vi "Query (Dynamic) 2.vi"(5 "Use VISA? (not visa GPIB only)":bool, 6 "Path Only":bool, 7 "Comms Layer":T1, 8 "error in":errorcluster, 9 "byte count":u32=4096 caption="byte count (4096)", 10 "Command":string, 11 "Comms":refnum<visa-resource-name>) -> (0 "error out":errorcluster, 2 "Response":string, 3 "Comms out":refnum<visa-resource-name>, 4 "path":path)   [LabVIEW 2013]
uses:
  <instrlib>/Mercury iXX/Public/Controls/Comms Transport Layer.ctl
  <vilib>/Instr/_visa.llb/VISA Flush IO Buffer Mask.ctl
  <instrlib>/Mercury iXX/Mercury iXX.lvlib
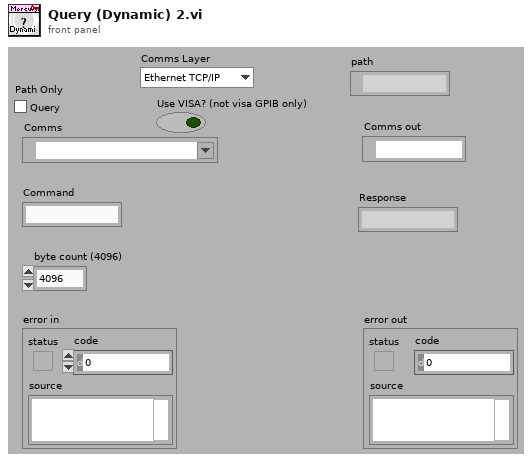
[diagram p1: front panel]
types:
  T1 = typedef "Mercury iXX.lvlib/Comms Transport Layer.ctl" = enum16{"Ethernet TCP/IP", "USB", "ISOBus - RS-232", "GPIB"}
  T2 = typedef "VISA Flush IO Buffer Mask.ctl" = u16
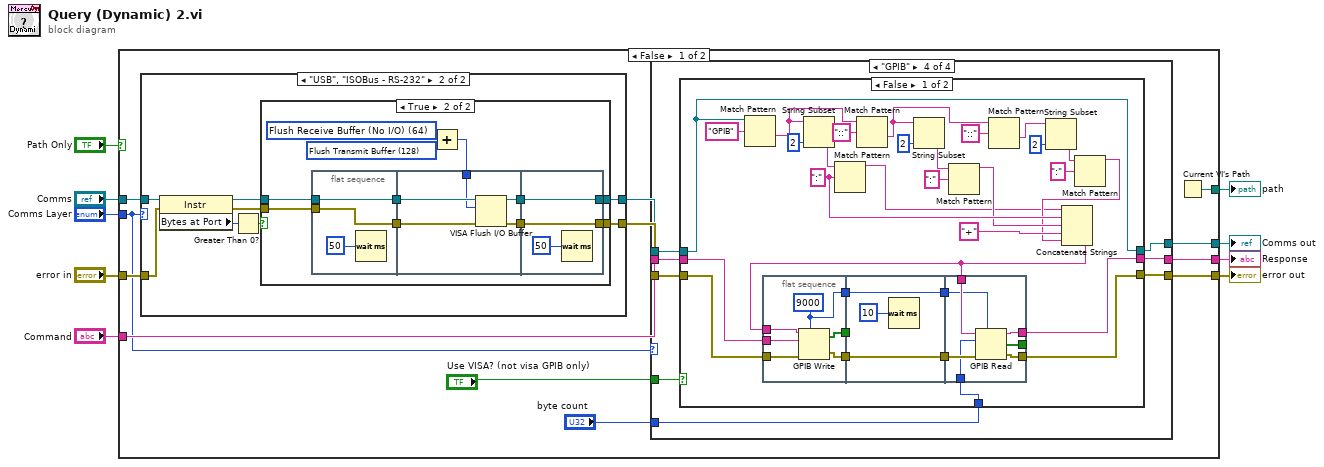
[diagram p0: block diagram]
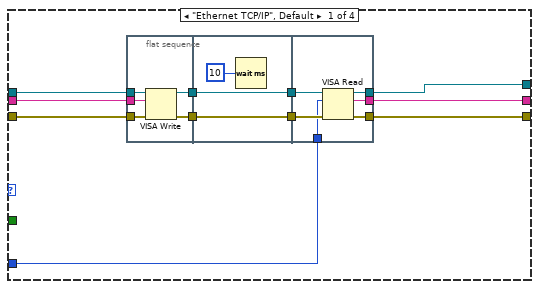
[diagram p2: hidden frame]
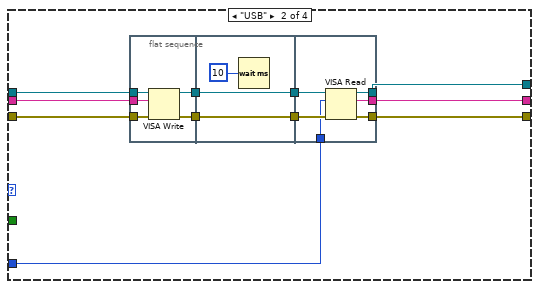
[diagram p3: hidden frame]
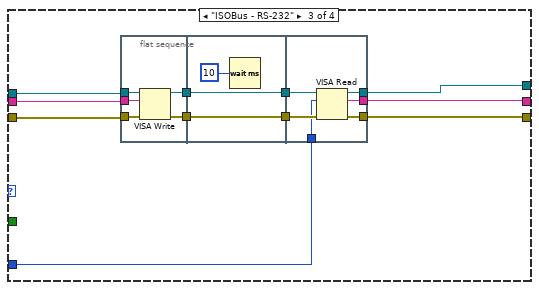
[diagram p4: hidden frame]
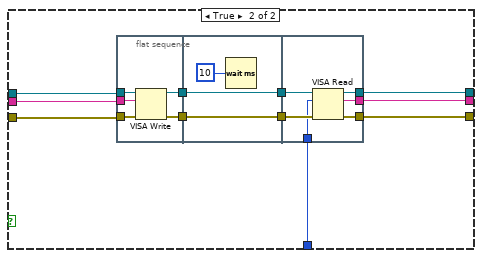
[diagram p5: hidden frame]
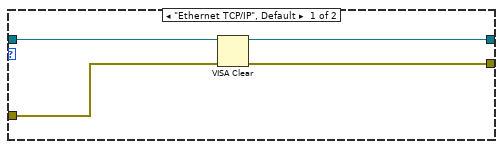
[diagram p6: hidden frame]
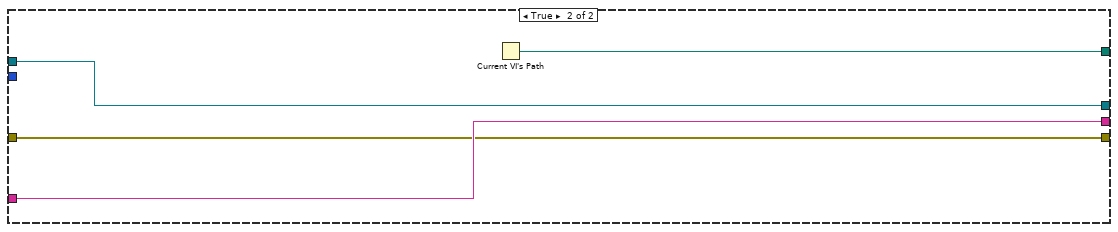
[diagram p8: hidden frame]
diagram:
  n1 = case shown="False" "Path Only" {
    tunnel: [w12 w215] -> w9
    tunnel: "Command" -> [w20 w215]
    tunnel: [w19 w216] -> w7
    tunnel: "error in" -> [w18 w214]
    tunnel: [w16 w214] -> w5
    tunnel: "Comms Layer" -> [w11 _]
    tunnel: "Comms" -> [w15 w216]
    tunnel: [w13 w213] -> w1
    frame False {
      n2 = case shown="\"USB\", \"ISOBus - RS-232\"" w11 {
        tunnel: w18 -> [w180 w187]
        tunnel: [w179 w181] -> w17
        tunnel: w15 -> [w178 w188]
        tunnel: [w177 w183] -> w14
        frame "Ethernet TCP/IP", Default {
          n3 = VISA Clear(VISA resource name=w178, error in (no error)=w180) -> (VISA resource name out=w177:refnum<visa-resource-name>, error out=w179:errorcluster)
        }
        frame "USB", "ISOBus - RS-232" {
          n4 = property class="Instr"(reference=w188, error in=w187) -> (reference out=w184:refnum<visa-resource-name>, error out=w182:errorcluster, "Bytes at Port"=w186:u32)
          n5 = Greater Than 0?(x=w186) -> (x > 0?=w185:bool)
          n6 = case shown="True" w185 {
            tunnel: w184 -> [w190 w199]
            tunnel: [w190 w201] -> w183
            tunnel: w182 -> [w189 w197]
            tunnel: [w189 w194] -> w181
            frame False {
            }
            frame True {
              w192 = T2 128 items=["Flush Receive Buffer"=16, "Write Transmit Buffer to Device"=32, "Flush Receive Buffer (No I/O)"=64, "Flush Transmit Buffer"=128] ("Mask")
              w193 = T2 64 items=["Flush Receive Buffer"=16, "Write Transmit Buffer to Device"=32, "Flush Receive Buffer (No I/O)"=64, "Flush Transmit Buffer"=128] ("Mask")
              n7 = flat-sequence {
                tunnel: w199 -> [w203]
                tunnel: [w203] -> w198
                tunnel: w197 -> [w202]
                tunnel: [w202] -> w196
                tunnel: [w209] -> w200
                tunnel: w198 -> [w208]
                tunnel: w196 -> [w207]
                tunnel: [w206] -> w195
                tunnel: w191 -> [w205]
                tunnel: [w211] -> w201
                tunnel: w200 -> [w211]
                tunnel: w195 -> [w210]
                tunnel: [w210] -> w194
                frame #0 {
                  n8 = Wait (ms)(milliseconds to wait=u32 50) -> ()  [unwired: 1 out]
                }
                frame #1 {
                  n9 = VISA Flush I/O Buffer(VISA resource name=w208, mask (16)=w205, error in (no error)=w207) -> (VISA resource name out=w209:refnum<visa-resource-name>, error out=w206:errorcluster)
                }
                frame #2 {
                  n10 = Wait (ms)(milliseconds to wait=u32 50) -> ()  [unwired: 1 out]
                }
              }
              n11 = Add(x=w193, y=w192) -> (x+y=w191:T2)
            }
          }
        }
      }
      n12 = case shown="\"GPIB\"" w11 {
        tunnel: "byte count" -> [w25 w53 w75 w101]
        tunnel: w20 -> [w27 w52 w77 w103]
        tunnel: [w22 w51 w72 w100] -> w19
        tunnel: w17 -> [w26 w50 w76 w102]
        tunnel: [w24 w49 w74 w98] -> w16
        tunnel: w14 -> [w28 w48 w78 w104]
        tunnel: [w23 w47 w73 w99] -> w12
        tunnel: "Use VISA? (not visa GPIB only)" -> [_ _ _ w97]
        frame "Ethernet TCP/IP", Default {
          n13 = flat-sequence {
            tunnel: w28 -> [w34]
            tunnel: w27 -> [w35]
            tunnel: [w37] -> w32
            tunnel: [w36] -> w31
            tunnel: w26 -> [w33]
            tunnel: w32 -> [w39]
            tunnel: w31 -> [w38]
            tunnel: [w39] -> w30
            tunnel: [w38] -> w29
            tunnel: w30 -> [w46]
            tunnel: w29 -> [w45]
            tunnel: [w44] -> w24
            tunnel: w25 -> [w43]
            tunnel: [w42] -> w22
            tunnel: [w41] -> w23
            frame #0 {
              n14 = VISA Write(VISA resource name=w34, write buffer=w35, error in (no error)=w33) -> (VISA resource name out=w37:refnum<visa-resource-name>, error out=w36:errorcluster)  [unwired: 1 out]
            }
            frame #1 {
              n15 = Wait (ms)(milliseconds to wait=u32 10) -> ()  [unwired: 1 out]
            }
            frame #2 {
              n16 = VISA Read(VISA resource name=w46, byte count=w43, error in (no error)=w45) -> (VISA resource name out=w42:refnum<visa-resource-name>, read buffer=w41:string, error out=w44:errorcluster)  [unwired: 1 out]
            }
          }
        }
        frame "USB" {
          n17 = flat-sequence {
            tunnel: w48 -> [w59]
            tunnel: w52 -> [w60]
            tunnel: [w62] -> w57
            tunnel: [w61] -> w56
            tunnel: w50 -> [w58]
            tunnel: w57 -> [w64]
            tunnel: w56 -> [w63]
            tunnel: [w64] -> w55
            tunnel: [w63] -> w54
            tunnel: w55 -> [w71]
            tunnel: w54 -> [w70]
            tunnel: [w69] -> w49
            tunnel: w53 -> [w68]
            tunnel: [w67] -> w51
            tunnel: [w66] -> w47
            frame #0 {
              n18 = VISA Write(VISA resource name=w59, write buffer=w60, error in (no error)=w58) -> (VISA resource name out=w62:refnum<visa-resource-name>, error out=w61:errorcluster)  [unwired: 1 out]
            }
            frame #1 {
              n19 = Wait (ms)(milliseconds to wait=u32 10) -> ()  [unwired: 1 out]
            }
            frame #2 {
              n20 = VISA Read(VISA resource name=w71, byte count=w68, error in (no error)=w70) -> (VISA resource name out=w67:refnum<visa-resource-name>, read buffer=w66:string, error out=w69:errorcluster)  [unwired: 1 out]
            }
          }
        }
        frame "ISOBus - RS-232" {
          n21 = flat-sequence {
            tunnel: w78 -> [w84]
            tunnel: w77 -> [w85]
            tunnel: [w87] -> w82
            tunnel: [w86] -> w81
            tunnel: w76 -> [w83]
            tunnel: w82 -> [w89]
            tunnel: w81 -> [w88]
            tunnel: [w89] -> w80
            tunnel: [w88] -> w79
            tunnel: w80 -> [w96]
            tunnel: w79 -> [w95]
            tunnel: [w94] -> w74
            tunnel: w75 -> [w93]
            tunnel: [w92] -> w72
            tunnel: [w91] -> w73
            frame #0 {
              n22 = VISA Write(VISA resource name=w84, write buffer=w85, error in (no error)=w83) -> (VISA resource name out=w87:refnum<visa-resource-name>, error out=w86:errorcluster)  [unwired: 1 out]
            }
            frame #1 {
              n23 = Wait (ms)(milliseconds to wait=u32 10) -> ()  [unwired: 1 out]
            }
            frame #2 {
              n24 = VISA Read(VISA resource name=w96, byte count=w93, error in (no error)=w95) -> (VISA resource name out=w92:refnum<visa-resource-name>, read buffer=w91:string, error out=w94:errorcluster)  [unwired: 1 out]
            }
          }
        }
        frame "GPIB" {
          n25 = case shown="False" w97 {
            tunnel: w104 -> [w123 w158]
            tunnel: w103 -> [w132 w157]
            tunnel: w102 -> [w131 w156]
            tunnel: [w123 w155] -> w100
            tunnel: [w130 w154] -> w99
            tunnel: [w118 w153] -> w98
            tunnel: w101 -> [w129 w152]
            frame False {
              w112 = ":" ("regular expression")
              n26 = Match Pattern(string=w123, regular expression="GPIB") -> (after substring=w125:string)  [unwired: 1 in, 3 out]
              n27 = flat-sequence {
                tunnel: [w141] -> w135
                tunnel: [w140] -> w134
                tunnel: w132 -> [w139]
                tunnel: w131 -> [w138]
                tunnel: w108 -> [w137]
                tunnel: [w136] -> w105
                tunnel: w135 -> [_]
                tunnel: w134 -> [w143]
                tunnel: [w143] -> w133
                tunnel: [w142] -> w106
                tunnel: w105 -> [w142]
                tunnel: w133 -> [w151]
                tunnel: [w150] -> w118
                tunnel: [w149] -> w130
                tunnel: [w148] -> _
                tunnel: w129 -> [w147]
                tunnel: w108 -> [w146]
                tunnel: w106 -> [w145]
                frame #0 {
                  w136 = 9000 ("timeout ms (488.2 global)")
                  n28 = GPIB Write(0:w137, 1:w139, 3:w138, 4:w136) -> (5:w141:bool[], 6:w140:errorcluster)  [unwired: 1 in]
                }
                frame #1 {
                  n29 = Wait (ms)(milliseconds to wait=u32 10) -> ()  [unwired: 1 out]
                }
                frame #2 {
                  n30 = GPIB Read(0:w146, 1:w147, 3:w151, 4:w145) -> (5:w149:string, 6:w148:bool[], 7:w150:errorcluster)  [unwired: 1 in]
                }
              }
              n31 = String Subset(string=w125, length (rest)=2 ("length (rest)")) -> (substring=w117:string)  [unwired: 1 in]
              n32 = Match Pattern(string=w117, regular expression=w112) -> (before substring=w107:string)  [unwired: 1 in, 3 out]
              n33 = Match Pattern(string=w125, regular expression="::") -> (after substring=w120:string)  [unwired: 1 in, 3 out]
              n34 = String Subset(string=w120, length (rest)=2 ("length (rest)")) -> (substring=w113:string)  [unwired: 1 in]
              n35 = Match Pattern(string=w113, regular expression=":") -> (before substring=w111:string)  [unwired: 1 in, 3 out]
              n36 = Match Pattern(string=w120, regular expression="::") -> (after substring=w121:string)  [unwired: 1 in, 3 out]
              n37 = String Subset(string=w121, length (rest)=2 ("length (rest)")) -> (substring=w114:string)  [unwired: 1 in]
              n38 = Match Pattern(string=w114, regular expression=":") -> (before substring=w109:string)  [unwired: 1 in, 3 out]
              n39 = Concatenate Strings(w107, w112, w111, "+" ("string"), w109) -> (w108:string)
            }
            frame True {
              n40 = flat-sequence {
                tunnel: w158 -> [w164]
                tunnel: w157 -> [w165]
                tunnel: [w167] -> w162
                tunnel: [w166] -> w161
                tunnel: w156 -> [w163]
                tunnel: w162 -> [w169]
                tunnel: w161 -> [w168]
                tunnel: [w169] -> w160
                tunnel: [w168] -> w159
                tunnel: w160 -> [w176]
                tunnel: w159 -> [w175]
                tunnel: [w174] -> w153
                tunnel: w152 -> [w173]
                tunnel: [w172] -> w155
                tunnel: [w171] -> w154
                frame #0 {
                  n41 = VISA Write(VISA resource name=w164, write buffer=w165, error in (no error)=w163) -> (VISA resource name out=w167:refnum<visa-resource-name>, error out=w166:errorcluster)  [unwired: 1 out]
                }
                frame #1 {
                  n42 = Wait (ms)(milliseconds to wait=u32 10) -> ()  [unwired: 1 out]
                }
                frame #2 {
                  n43 = VISA Read(VISA resource name=w176, byte count=w173, error in (no error)=w175) -> (VISA resource name out=w172:refnum<visa-resource-name>, read buffer=w171:string, error out=w174:errorcluster)  [unwired: 1 out]
                }
              }
            }
          }
        }
      }
      n44 = Current VI's Path() -> (path=w13:path)
    }
    frame True {
      n45 = Current VI's Path() -> (path=w213:path)
    }
  }
  "Response" <- w9
  "error out" <- w5
  "Comms out" <- w7
  "path" <- w1
